vi "Check if PPL is Cached.vi"(8 "error in":errorcluster, 11 "PPL Details":T1) -> (0 "error out":errorcluster, 1 "Is Cached?":bool, 3 "Cache Path":path)   [LabVIEW 2020, in "ClassLoader.lvlib"]
doc: "Build cache path from PPL details and check if there is a file at the Cache Path."
uses:
  ClassLoader.lvlib
  Ctl/Ctl_PPL Details.ctl
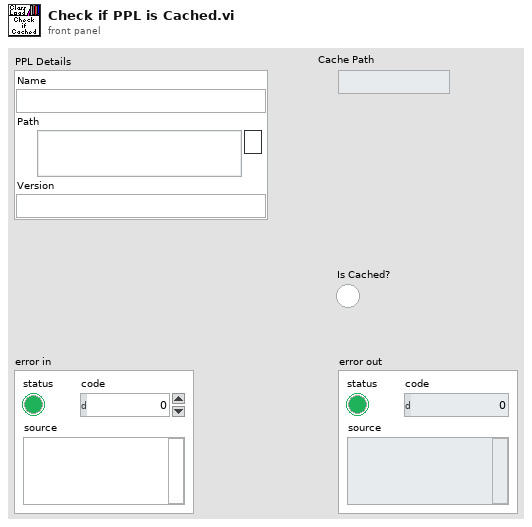
[diagram p1: front panel]
types:
  T1 = typedef "ClassLoader.lvlib/Ctl_PPL Details.ctl" = cluster{"Name":string, "Path":path, "Version":string}
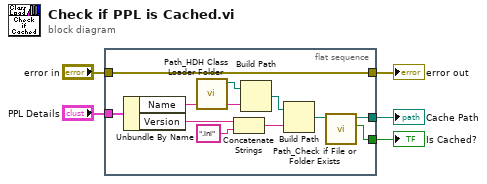
[diagram p0: block diagram]
diagram:
  n1 = flat-sequence {
    tunnel: "PPL Details" -> [w16]
    tunnel: [w8] -> w4
    tunnel: "error in" -> [w8]
    tunnel: [w7] -> w2
    tunnel: [w6] -> w1
    frame #0 {
      n2 = Unbundle By Name(w16) -> ("Name"=w14:string, "Version"=w12:string)
      n3 = call "Path_HDH Class Loader Folder.vi"() -> ("HDH\\Class Loader path"=w15:path)  [unwired: 11 in]
      n4 = Concatenate Strings(w12, ".ini" ("string")) -> (w10:string)
      n5 = Build Path(base path=w15, name or relative path=w14) -> (appended path=w13:path)
      n6 = Build Path(base path=w13, name or relative path=w10) -> (appended path=w9:path)
      n7 = call "Path_Check if File or Folder Exists.vi"("File or Folder Path in"=w9) -> ("File or Folder Found?"=w7:bool, "File or Folder Path dub"=w6:path)  [unwired: 9 in]
    }
  }
  "Is Cached?" <- w2
  "error out" <- w4
  "Cache Path" <- w1
